vi "VoltageQueue_Global.vi"() -> ()   [LabVIEW 2017]
uses:
  MessageQueue/QueueOperations/Message Cluster.ctl
  MessageQueue/MessageQueue.lvlib
panel:
  in  "Voltage":dbl
  in  "Message Queue":refnum<queue>
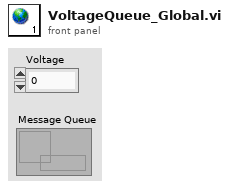
[diagram p1: front panel]
diagram:
